vi "Shutdown.vi"(11 "Application in":refnum<class "Application.lvclass">) -> (0 "error out":errorcluster, 3 "Application out":refnum<class "Application.lvclass">)   [LabVIEW 2017, in "Application.lvclass"]
doc: "Application.lvclass:Shutdown.vi does nothing. Child classes should override this VI with any work needed to quit the application. This includes releasing any resources acquired during Setup and writing any configuration files if options changed during the run of the application. \n\nThis VI will only be called if no error was returned from Setup, and it will still be called even if Execute returns an error."
uses:
  Application.lvclass
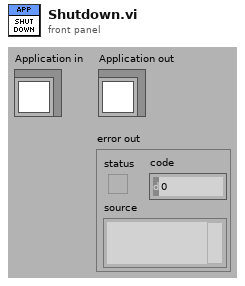
[diagram p1: front panel]
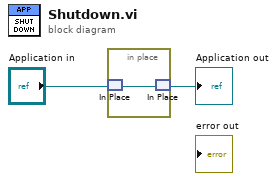
[diagram p0: block diagram]
diagram:
  n1 = in-place {
    n2 = in-place-match #1("Application in") -> (w3:refnum<class "Application.lvclass">)
    n3 = in-place-match #1(w3) -> (→"Application out":refnum<class "Application.lvclass">)
  }
